vi "Save_Before-After_Tracks-3.vi"(0 "[IN] Grouped tracks":T2(array[cluster]), 1 "[IN] Filtering Settings":T1, 2 "# channel":u8, 3 "[IN] AVI Refnum":T3, 5 "[IN] Tracks group":i32 min=0 max=498, 9 "Save movies?":bool, 11 "error IN":errorcluster, 12 "default name":string, 13 "[IN] FPS":u32, 14 "Keep Nega-\ntive Values?":bool) -> (15 "error OUT":errorcluster)   [LabVIEW 2013]
uses:
  <vilib>/vision/Avi.llb/IMAQ AVI2 Refnum.ctl
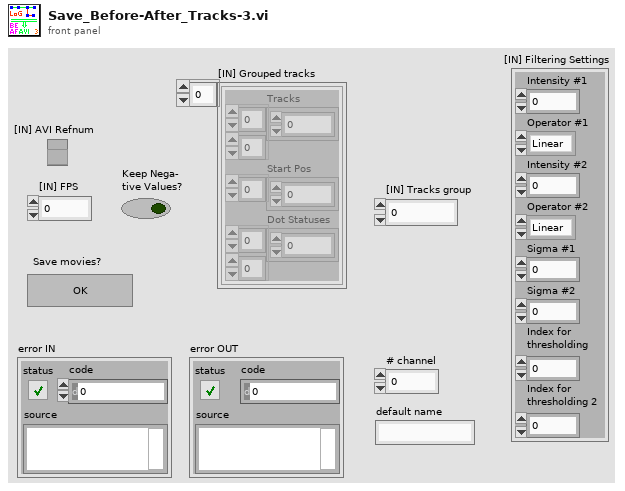
[diagram p1: front panel]
types:
  T1 = cluster{"Intensity #1":sgl, "Operator #1":enum32{"Linear", "Log", "Exp", "Square", "Square root", "Power X", "Power 1/X"}, "Intensity #2":sgl, "Operator #2":enum32{"Linear", "Log", "Exp", "Square", "Square root", "Power X", "Power 1/X"}, "Sigma #1":dbl, "Sigma #2":dbl, "Index for \nthresholding":u8, "Index for \nthresholding 2":u8}
  T2 = cluster{"Tracks":dbl[][], "Start Pos":i32[], "Dot Statuses":i16[][]}[]
  T3 = typedef "IMAQ AVI2 Refnum.ctl" = refnum<k20>
  T4 = typedef "Image Type" = u32
  T5 = typedef "IMAQ Image.ctl" = refnum<image>
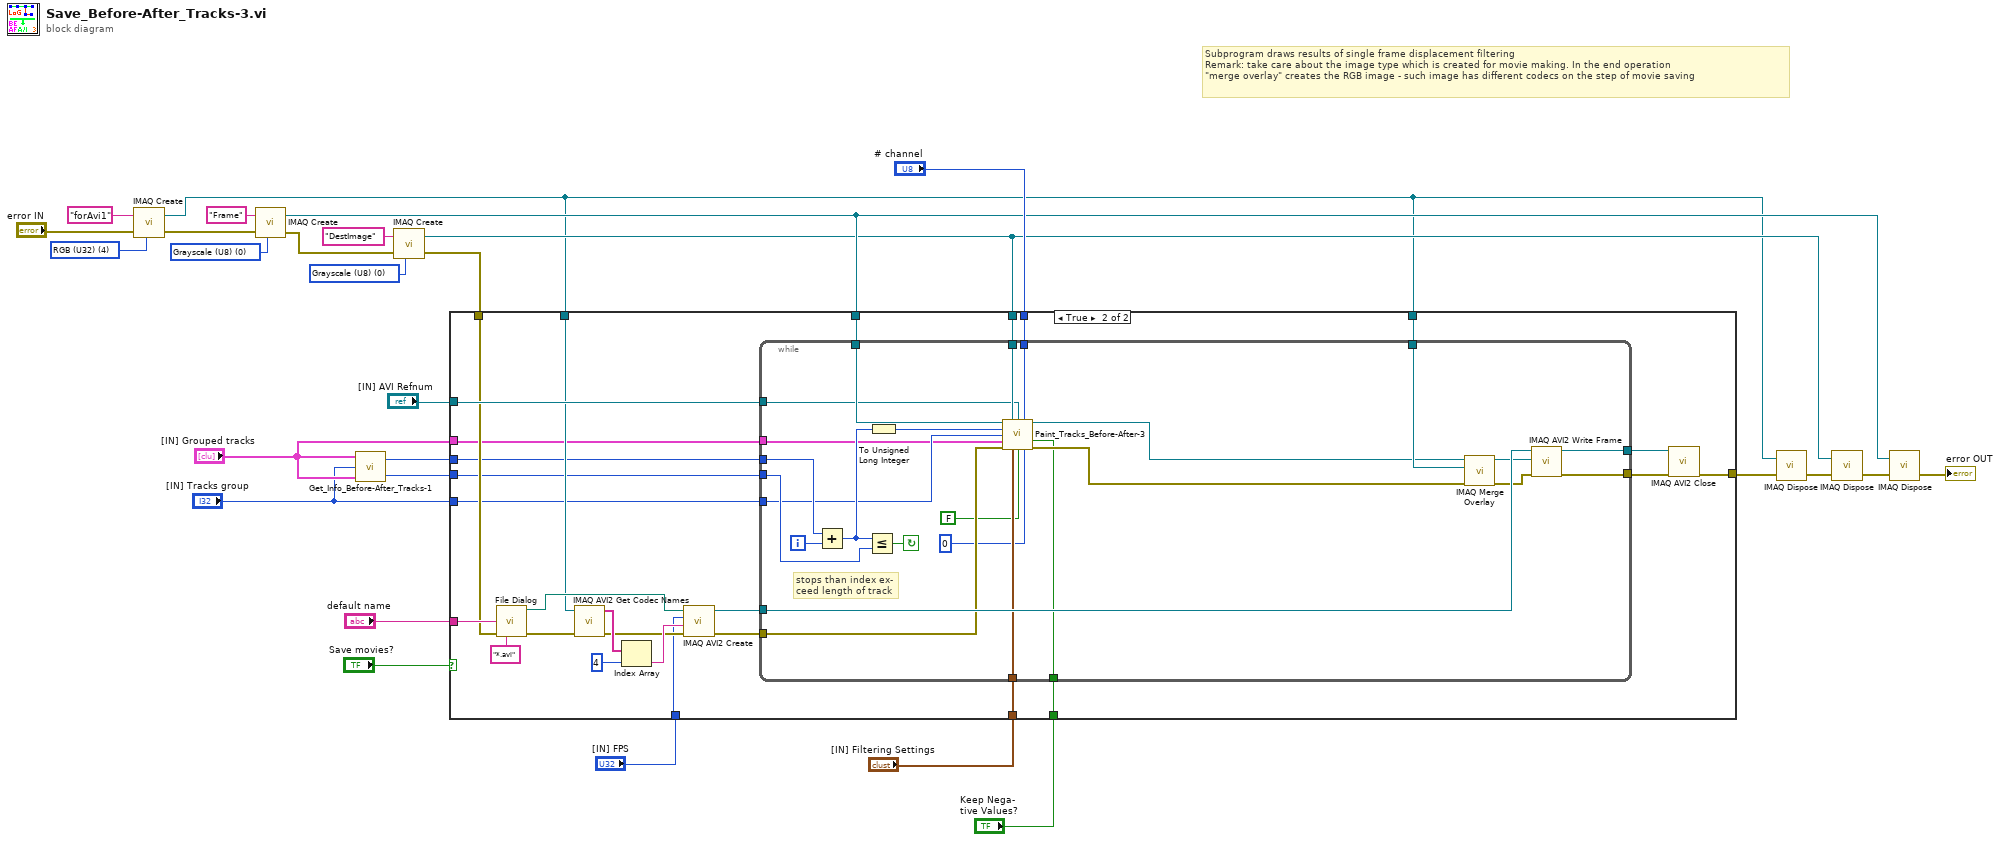
[diagram p0: block diagram]
diagram:
  w12 = T4 0 items=["Grayscale (U8)", "Grayscale (I16)", "Grayscale (SGL)", "Complex (CSG)", "RGB (U32)", "HSL (U32)", "RGB (U64)", "Grayscale (U16)"] ("Image Type")
  w20 = T4 0 items=["Grayscale (U8)", "Grayscale (I16)", "Grayscale (SGL)", "Complex (CSG)", "RGB (U32)", "HSL (U32)", "RGB (U64)", "Grayscale (U16)"] ("Image Type")
  w17 = T4 4 items=["Grayscale (U8)", "Grayscale (I16)", "Grayscale (SGL)", "Complex (CSG)", "RGB (U32)", "HSL (U32)", "RGB (U64)", "Grayscale (U16)"] ("Image Type")
  # "Subprogram draws results of single frame displacement filtering\nRemark: take care about the image type which is created for movie making. In the end operation\n\"merge overlay\" creates the RGB image - such image has different codecs on the step of movie saving"
  n1 = call "IMAQ Create"("Image Name"="forAvi1", "Image Type"=w17, "error in (no error)"="error IN") -> ("New Image"=w3:T5, "error out"=w16:errorcluster)  [unwired: 2 in]
  n2 = call "IMAQ Create"("Image Name"="Frame", "Image Type"=w20, "error in (no error)"=w16) -> ("New Image"=w6:T5, "error out"=w10:errorcluster)  [unwired: 2 in]
  n3 = call "Get_Info_Before-After_Tracks-1.vi"("[IN] After Tracks"="[IN] Grouped tracks", "[IN] Tracks group"="[IN] Tracks group", "[IN] Before Tracks"="[IN] Grouped tracks") -> ("Maximal Frame\n(finish point all\ntracks)"=w14:i32, "[OUT] Min Start Pos"=w15:i32)
  n4 = call "IMAQ Create"("Image Name"="DestImage", "Image Type"=w12, "error in (no error)"=w10) -> ("New Image"=w4:T5, "error out"=w9:errorcluster)  [unwired: 2 in]
  n5 = case shown="True" "Save movies?" {
    tunnel: w3 -> [_ w40]
    tunnel: "[IN] FPS" -> [_ w49]
    tunnel: "[IN] AVI Refnum" -> [_ w48]
    tunnel: [w29 w44] -> w22
    tunnel: "default name" -> [_ w46]
    tunnel: w9 -> [w29 w42]
    tunnel: w15 -> [_ w39]
    tunnel: w14 -> [_ w38]
    tunnel: "[IN] Grouped tracks" -> [_ w37]
    tunnel: w6 -> [_ w36]
    tunnel: w4 -> [_ w35]
    tunnel: "[IN] Tracks group" -> [_ w34]
    tunnel: "# channel" -> [_ w33]
    tunnel: w3 -> [_ w32]
    tunnel: "[IN] Filtering Settings" -> [_ w31]
    tunnel: "Keep Nega-\ntive Values?" -> [_ w30]
    frame False {
    }
    frame True {
      n6 = call "File Dialog"("default name"=w46, "error in"=w42, "pattern (all files)"="*.avi") -> ("selected path"=w50:path, "error out"=w47:errorcluster)  [unwired: 9 in, 2 out]
      n7 = call "IMAQ AVI2 Get Codec Names"("error in (no error)"=w47, "Image"=w40) -> ("error out"=w54:errorcluster, "Codec Names"=w56:string[])  [unwired: 8 in]
      n8 = Index Array(array=w56, index=4) -> (element=w55:string)
      n9 = call "IMAQ AVI2 Create"("error in (no error)"=w54, "Codec"=w55, "Frames Per Second"=w49, "AVI Path"=w50) -> ("error out"=w53:errorcluster, "AVI Refnum"=w52:T3)  [unwired: 6 in]
      n10 = while {
        tunnel: w48 -> [w64]
        tunnel: w53 -> [w66]
        tunnel: w52 -> [w81]
        tunnel: [w79] -> w45
        tunnel: [w80] -> w43
        tunnel: w39 -> [w75]
        tunnel: w38 -> [w77]
        tunnel: w37 -> [w67]
        tunnel: w36 -> [w70]
        tunnel: w35 -> [w65]
        tunnel: w34 -> [w68]
        tunnel: w33 -> [w63]
        tunnel: w32 -> [w71]
        tunnel: w31 -> [w60]
        tunnel: w30 -> [w57]
        i -> [w78]
        stop <- w76 continue-if-true
        # "stops than index ex-\nceed length of track"
        n11 = Add(x=w75, y=w78) -> (x+y=w72:i32)
        n12 = Less Or Equal?(x=w72, y=w77) -> (x <= y?=w76:bool)
        n13 = To Unsigned Long Integer(number=w72) -> (unsigned 32bit integer=w69:u32)
        n14 = call "Paint_Tracks_Before-After-3.vi"("[IN] Frame"=w70, "[IN] Destina\ntion Image"=w65, "[IN] AVI Refnum"=w64, "[IN] # channel"=w63, "[IN] Testing Frame"=w69, "[IN] Tracks group"=w68, "[IN] Grouped Tracks"=w67, "Keep Nega-\ntive Values?"=w57, "error IN"=w66, "[IN] Filtering Settings"=w60, "[IN] Delete Tracs"=FALSE, "[IN] Additional Index"=0) -> ("[OUT] Image with\nDisplacements"=w62:T5, "error OUT"=w61:errorcluster)  [unwired: 2 in]
        n15 = call "IMAQ Merge Overlay"("error in (no error)"=w61, "Image Dst"=w71, "Image Src"=w62) -> ("error out"=w73:errorcluster, "Image Dst Out"=w74:T5)  [unwired: 7 in]
        n16 = call "IMAQ AVI2 Write Frame"("error in (no error)"=w73, "Image"=w74, "AVI Refnum"=w81) -> ("error out"=w79:errorcluster, "AVI Refnum (duplicate)"=w80:T3)  [unwired: 6 in, 1 out]
      }
      n17 = call "IMAQ AVI2 Close"("error in (no error)"=w45, "AVI Refnum"=w43) -> ("error out"=w44:errorcluster)  [unwired: 9 in]
    }
  }
  n18 = call "IMAQ Dispose"("Image"=w3, "error in (no error)"=w22) -> ("error out"=w21:errorcluster)  [unwired: 4 in]
  n19 = call "IMAQ Dispose"("Image"=w4, "error in (no error)"=w21) -> ("error out"=w18:errorcluster)  [unwired: 4 in]
  n20 = call "IMAQ Dispose"("Image"=w6, "error in (no error)"=w18) -> ("error out"=→"error OUT":errorcluster)  [unwired: 4 in]
